vi "LIA Example FPGA.vi"() -> ()   [LabVIEW 2017]
uses:
  <instrlib>/_niInstr/Streaming/v1/Common/Stream State.ctl
  <instrlib>/_niInstr/Data Trigger/v1/Shared/Public/Edge Configuration FXP(+-,18,1).ctl
  <instrlib>/_niInstr/Data Trigger/v1/Shared/Public/Edge Configuration Trigger Slope.ctl
  <vilib>/Platform/TimedLoop/XDataNode/timing_clust.ctl
  <vilib>/Platform/TimedLoop/XDataNode/nitl_modes.ctl
  <vilib>/Platform/TimedLoop/XDataNode/wakeup.ctl
  <instrlib>/_niInstr/DSP/v1/Shared/Public/IQ Data.ctl
  <vilib>/rvi/Emulation/niFpgaSctlEmulationGetInTimedLoop.vi
  <vilib>/rvi/Emulation/niFpgaEmulationReportErrorSimple.vi
  <vilib>/rvi/Emulation/niFpgaGetClockAttributes.vi
  <vilib>/rvi/Emulation/niFpgaCriticalErrorInLSC.vi
  <instrlib>/_niInstr/DSP/v1/FPGA/Public/Sub VIs/Frequency Shift/Frequency Shift - 1 spc.vi
  <userlib>/_NI Noise Generation IP/FPGA/Public/Low Level/AWGN FXP23x2.vi
  <instrlib>/_niInstr/DSP/v1/FPGA/Public/Sub VIs/Frequency Shift/Frequency Shift - 2 spc.vi
  <vilib>/rvi/eio/common/nirviEmuTemplateMethod_errors.vi
  <vilib>/Platform/TimedLoop/XDataNode/XDataNode.xnode
  <instrlib>/_niInstr/DSP/v1/Xnodes/Public/Frequency Shift/niInstr DSP v1 Frequency Shift FPGA.xnode
  <vilib>/rvi/FXPMathLib/FxpMul/XNode/nifxpmath_Multiplier.xnode
  <vilib>/rvi/FXPMathLib/FxpAdd/XNode/nifxpmath_Add.xnode
  <vilib>/eio/EIONode/EIONode.xnode
  <vilib>/Platform/TimedLoop/XDataNode/XDNodeRunTimeDep.lvlib
  <instrlib>/_niInstr/Basic Elements/v1/FPGA/niInstr Basic Elements v1 FPGA.lvlib
  <instrlib>/_niInstr/DSP/v1/Shared/niInstr DSP v1 Shared.lvlib
  <instrlib>/_niInstr/DSP/v1/FPGA/niInstr DSP v1 FPGA.lvlib
  Program Files (x86)/National Instruments/LabVIEW 2017/examples/Lock-In Amplifier/lib/fpga/Lock-In Amplifier Example FPGA.lvlib
  <instrlib>/_niInstr/Streaming/v1/Common/niInstr Streaming v1 Common.lvlib
  <userlib>/_NI Noise Generation IP/FPGA/NI Noise Generation IP FPGA v2.lvlib
  <vilib>/rvi/FXPMathLib/sim/FxpSim.dll
  <instrlib>/_niInstr/Data Trigger/v1/Shared/niInstr Data Trigger v1 Shared.lvlib
panel:
  in  "pll.digital config 1":T1
  in  "pll.digital config 0":T1
  in  "pll.m 0":i8
  in  "pll.m 1":i8
  in  "pll.q 1":fxp<+/-,48,0>
  in  "pll.q 0":fxp<+/-,48,0>
  in  "lock-in.enable 3":bool
  in  "lock-in.enable 2":bool
  in  "lock-in.enable 1":bool
  in  "lock-in.carrier 3":fxp<+/-,48,0>
  in  "lock-in.carrier 2":fxp<+/-,48,0>
  in  "lock-in.enable 0":bool
  in  "lock-in.channel select 3":i32
  in  "lock-in.carrier select 3":i32
  in  "lock-in.cic config valid 3":bool
  in  "lock-in.cic config 3":cluster{"factor":fxp<+,16,16>, "shift":i16}
  in  "lock-in.reset 3":bool
  out "stream.state 3":T3 caption="stream.state 0"
  out "stream.samples transferred 3":u64 caption="stream.samples transferred 0"
  out "stream.metadata 3":u64 caption="stream.metadata 0"
  in  "stream.num samples 3":u64 caption="stream.num samples 0"
  in  "stream.request state 3":T3 caption="stream.request state 0"
  in  "lock-in.channel select 2":i32
  in  "lock-in.carrier select 2":i32
  in  "lock-in.cic config valid 2":bool
  in  "lock-in.cic config 2":cluster{"factor":fxp<+,16,16>, "shift":i16}
  in  "lock-in.reset 2":bool
  out "stream.state 2":T3 caption="stream.state 0"
  out "stream.samples transferred 2":u64 caption="stream.samples transferred 0"
  out "stream.metadata 2":u64 caption="stream.metadata 0"
  in  "stream.num samples 2":u64 caption="stream.num samples 0"
  in  "stream.request state 2":T3 caption="stream.request state 0"
  out "pll.vco output 0":fxp<+/-,48,0> format="%.49g"
  out "pll.vco output 1":fxp<+/-,48,0> format="%.49g"
  out "stream.metadata 4":u64 caption="stream.metadata 0"
  out "stream.samples transferred 4":u64 caption="stream.samples transferred 0"
  out "stream.state 4":T3 caption="stream.state 0"
  in  "stream.request state 4":T3 caption="stream.request state 0"
  in  "stream.num samples 4":u64 caption="stream.num samples 0"
  in  "preview.channel select":i32
  in  "ao.reset 3":bool
  in  "ao.carrier 2":fxp<+/-,48,0>=0.010000000000001563
  in  "ao.level 2":fxp<+/-,18,1>
  in  "ao.reset 2":bool
  in  "ao.carrier 1":fxp<+/-,48,0>=0.010000000000001563
  in  "ao.level 1":fxp<+/-,18,1>
  in  "ao.reset 1":bool
  in  "ao.reset 0":bool
  in  "ao.carrier 0":fxp<+/-,48,0>=0.010000000000001563
  in  "ao.level 0":fxp<+/-,18,1>
  in  "lock-in.channel select 1":i32
  in  "lock-in.channel select 0":i32
  in  "stream.request state 1":T3 caption="stream.request state 0"
  in  "stream.num samples 1":u64 caption="stream.num samples 0"
  out "stream.metadata 1":u64 caption="stream.metadata 0"
  out "stream.samples transferred 1":u64 caption="stream.samples transferred 0"
  out "stream.state 1":T3 caption="stream.state 0"
  in  "lock-in.reset 1":bool
  in  "lock-in.cic config 1":cluster{"factor":fxp<+,16,16>, "shift":i16}
  in  "lock-in.cic config valid 1":bool
  in  "lock-in.carrier select 1":i32
  in  "lock-in.carrier select 0":i32
  in  "lock-in.cic config valid 0":bool
  in  "lock-in.cic config 0":cluster{"factor":fxp<+,16,16>, "shift":i16}
  in  "lock-in.reset 0":bool
  in  "lock-in.carrier 1":fxp<+/-,48,0>
  in  "lock-in.carrier 0":fxp<+/-,48,0>
  in  "ao.level 3":fxp<+/-,18,1>
  in  "pll.channel 1":i32
  in  "pll.reset 1":bool
  in  "pll.enable 1":bool
  in  "pll.channel 0":i32
  in  "ao.noise gain 3":fxp<+,18,1>=0.01000213623046875
  in  "ao.carrier 3":fxp<+/-,48,0>=0.010000000000001563
  in  "ao.noise seeds 3":fxp<+,23,23>[](array[numeric])=[1.0, 12323.0]
  in  "pll.reset 0":bool
  in  "pll.enable 0":bool
  in  "stream.request state 0":T3
  in  "stream.num samples 0":u64
  out "stream.metadata 0":u64
  out "stream.samples transferred 0":u64
  out "stream.state 0":T3
  out "IO Module\\InitDone":bool
  out "IO Module\\User Error":u32
  in  "IO Module\\User Command":u32
  in  "IO Module\\User Command Valid":bool
  out "IO Module\\User Command Ready":bool
  in  "IO Module\\User Command Arg 0":u32
  in  "IO Module\\User Command Arg 1":u32
  out "IO Module\\User Command Error":u16
  out "IO Module\\User Command Return":u32
  out "IO Module\\User Command Return Valid":bool
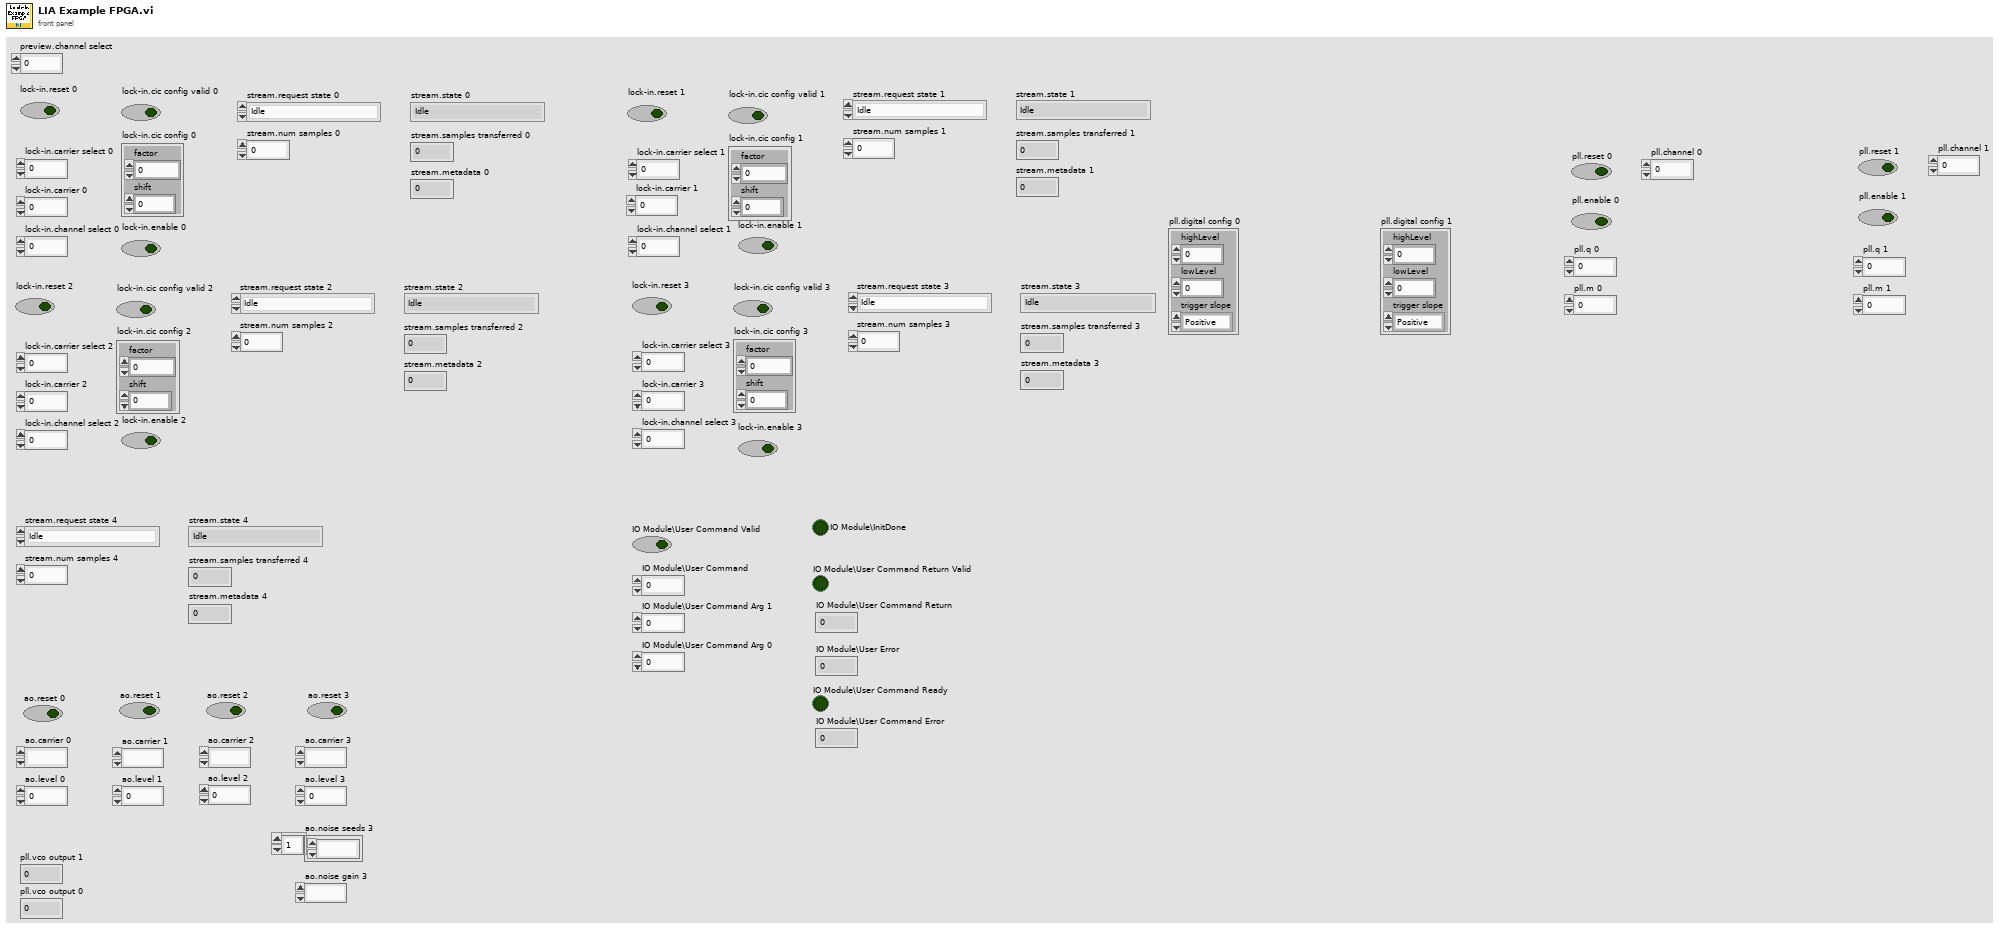
[diagram p1: front panel]
types:
  T1 = typedef "niInstr Data Trigger v1 Shared.lvlib/Edge Configuration FXP(+-,18,1).ctl" = cluster{"highLevel":fxp<+/-,18,1>, "lowLevel":fxp<+/-,18,1>, "trigger slope":T2}
  T2 = typedef "niInstr Data Trigger v1 Shared.lvlib/Edge Configuration Trigger Slope.ctl" = enum8{"Positive", "Negative"}
  T3 = typedef "niInstr Streaming v1 Common.lvlib/Stream State.ctl" = enum8{"Idle", "Finite Transfer", "Continuous", "Done", "Error", "Not Ready", "Cancel"}
  T4 = typedef "XDNodeRunTimeDep.lvlib/timing_clust.ctl" = cluster{"Expected End [f-1]":u64, "Actual End [f-1]":u64, "Finished Late? [f-1]":bool, "Expected End [i-1]":u64, "Actual End [i-1]":u64, "Finished Late? [i-1]":bool, "Expected Start [i]":u64, "Actual Start [i]":u64, "Expected Start [f]":u64, "Actual Start [f]":u64, "Source Name":string, "Structure Name":string, "Period":i64, "Deadline":i64, "Offset":i64, "Start":i64, "Priority":i32, "Timeout":i32, "Mode":T5, "Wakeup Reason":T6, "Error":errorcluster, "Source Type":string, "Secondary Source Type":string, "Global End Time":u64, "Global Start Time":u64, "Frame Duration":u64, "Iteration Duration":u64, "Assigned CPU":i32, "I/O Scan Engine Mode":u32}
  T5 = typedef "XDNodeRunTimeDep.lvlib/nitl_modes.ctl" = enum32{"No Change", "Process missed periods, maintain original phase", "Discard missed periods, maintain original phase", "Process missed periods, ignore original phase", "Discard missed periods, ignore original phase"}
  T6 = typedef "XDNodeRunTimeDep.lvlib/wakeup.ctl" = enum32{"Normal", "Aborted", "Asynchronous wakeup", "Timing source error", "Timed loop error", "Timeout"}
  T7 = cluster{"stream.num samples 0":u64, "stream.request state 0":T3, "stream.index 0":i16}
  T8 = typedef "niInstr DSP v1 Shared.lvlib/IQ Data.ctl" = cluster{"I":fxp<+/-,18,1>, "Q":fxp<+/-,18,1>, "overflow":bool}
  T9 = cluster{"stream.metadata 0":u64, "stream.samples transferred 0":u64, "stream.state 0":T3}
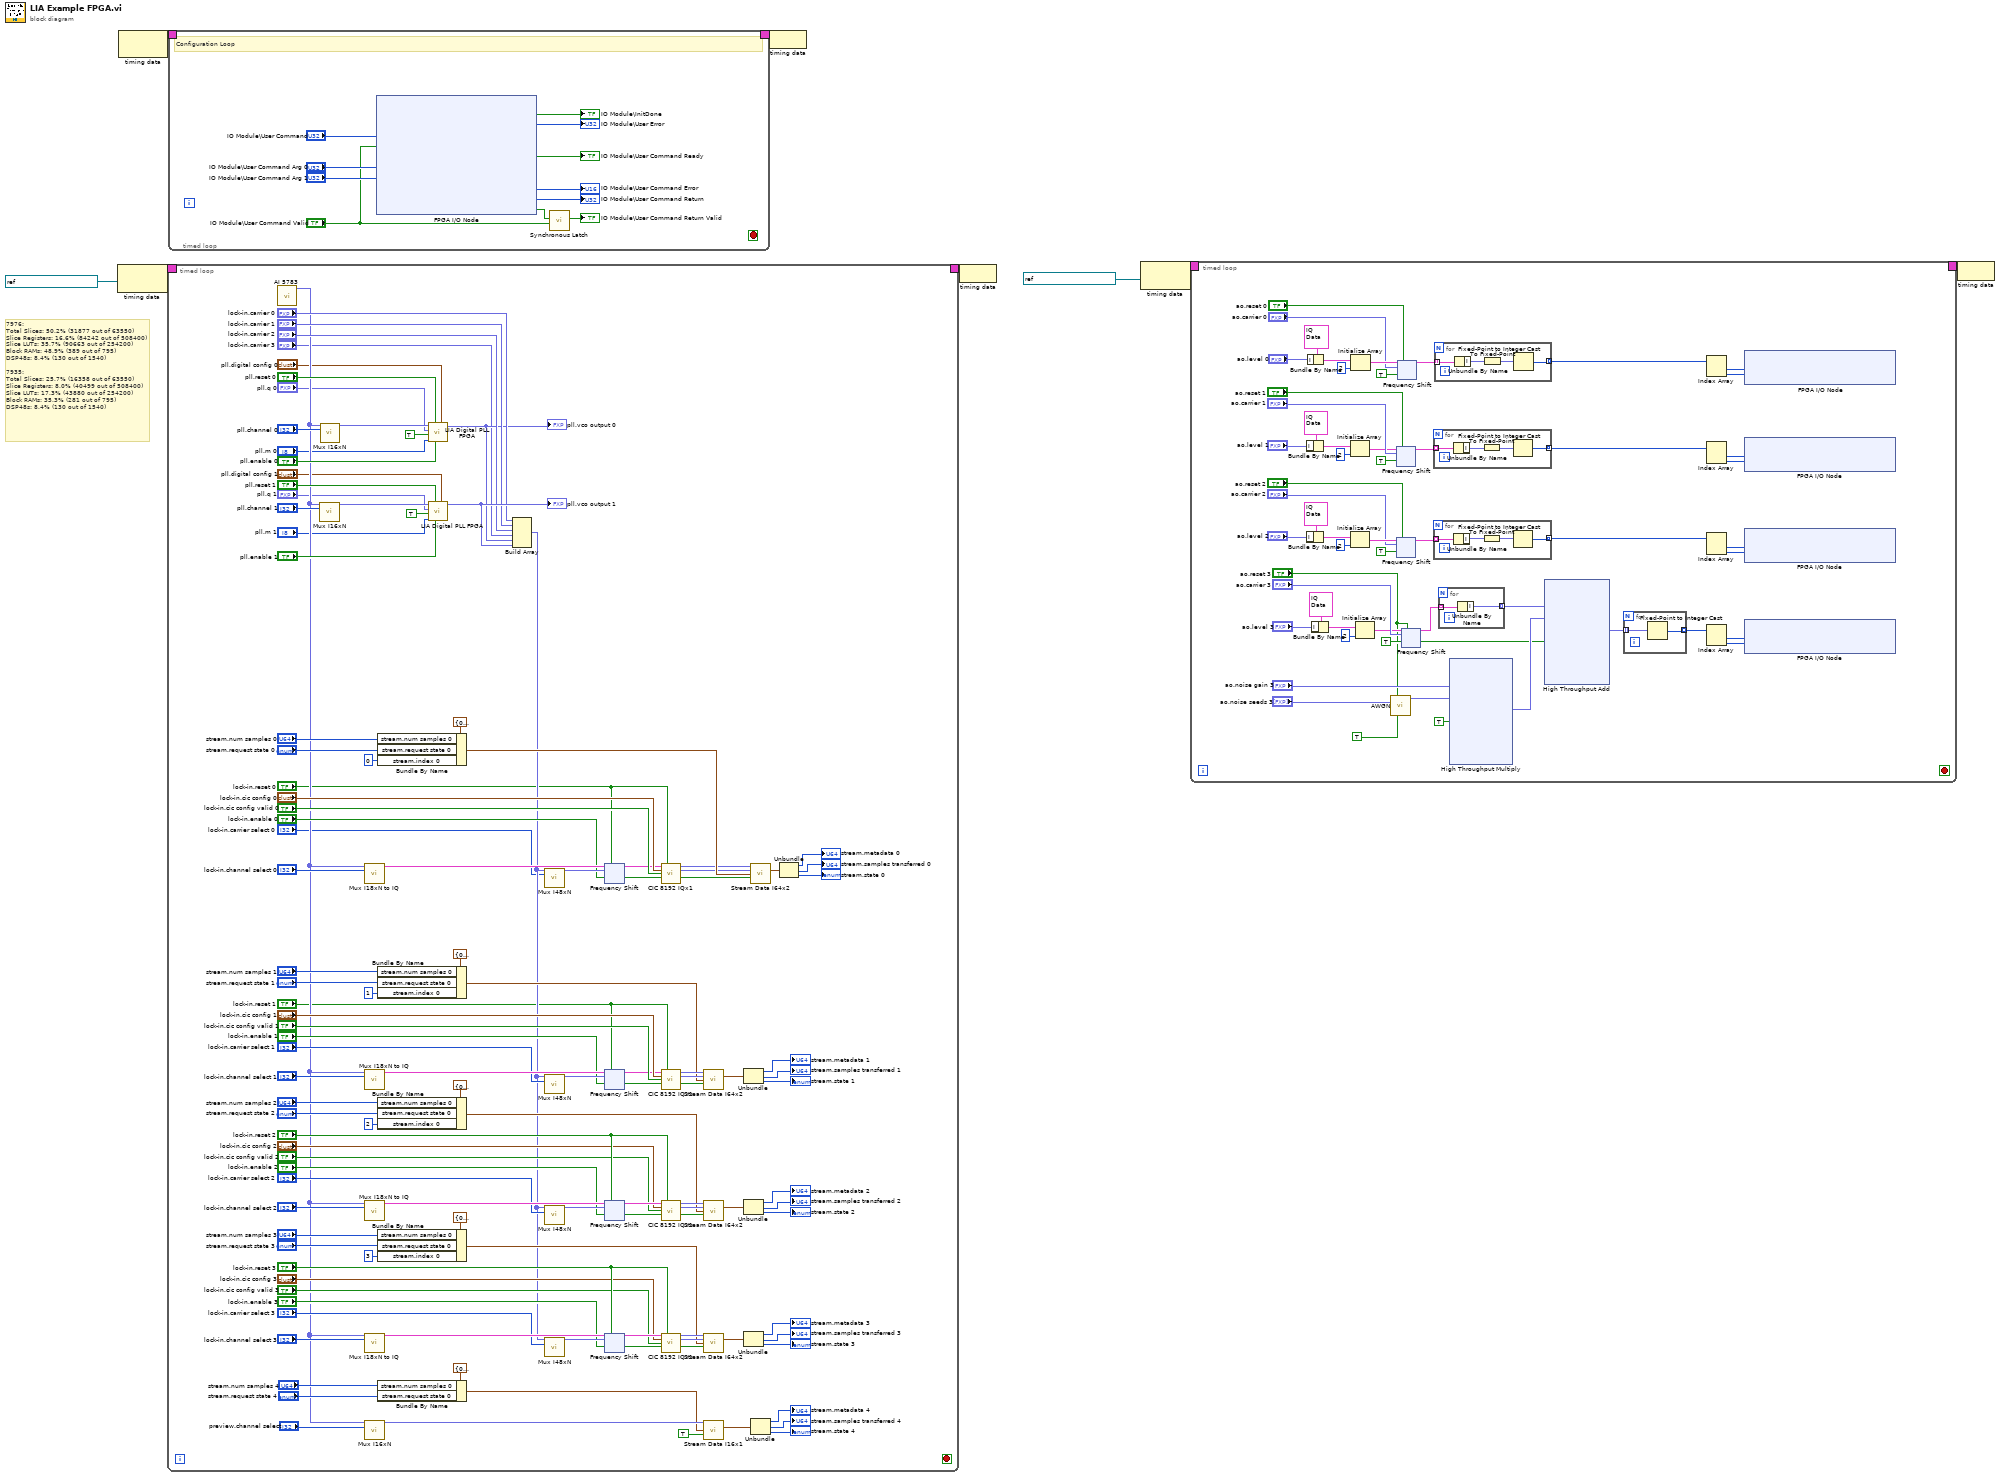
[diagram p0: block diagram]
diagram:
  # "7976:\nTotal Slices: 50.2% (31877 out of 63550)\nSlice Registers: 16.6% (84242 out of 508400)\nSlice LUTs: 35.7% (90663 out of 254200)\nBlock RAMs: 48.9% (389 out of 795)\nDSP48s: 8.4% (130 out of 1540)\n\n7935:\nTotal Slices: 25.7% (16358 out of 63550)\nSlice Registers: 8.0% (40499 out of 508400)\nSlice LUTs: 17.3% (43880 out of 254200)\nBlock RAMs: 35.3% (281 out of 795)\nDSP48s: 8.4% (130 out of 1540)"
  n1 = node-c288(refnum<k21> "IO Module\\Data Clock" ("Source Name")) -> (w8:T4)
  n2 = node-c288() -> (w2:T4)  [unwired: 1 in]
  n3 = timed-loop {
    timing: w8 -> [_]
    timing-out: [_] -> w7
    stop <- _ stop-if-true
    n4 = call "AI 5783.vi"() -> ("i18x1"=w27:fxp<+/-,18,1>[])  [unwired: 14 in, 1 out]
    n5 = call "Mux I16xN.vi"("i16xn in"=w27, "index"="pll.channel 1") -> ("i16 out"=w30:fxp<+/-,18,1>)  [unwired: 12 in, 1 out]
    n6 = call "Mux I16xN.vi"("i16xn in"=w27, "index"="pll.channel 0") -> ("i16 out"=w129:fxp<+/-,18,1>)  [unwired: 12 in, 1 out]
    n7 = call "Mux I18xN to IQ.vi"("i16xn in"=w27, "index"="lock-in.channel select 0") -> ("output"=w124:T8)  [unwired: 12 in, 1 out]
    n8 = call "Mux I18xN to IQ.vi"("i16xn in"=w27, "index"="lock-in.channel select 1") -> ("output"=w110:T8)  [unwired: 12 in, 1 out]
    n9 = call "Mux I18xN to IQ.vi"("i16xn in"=w27, "index"="lock-in.channel select 2") -> ("output"=w81:T8)  [unwired: 12 in, 1 out]
    n10 = call "Mux I18xN to IQ.vi"("i16xn in"=w27, "index"="lock-in.channel select 3") -> ("output"=w60:T8)  [unwired: 12 in, 1 out]
    n11 = call "Mux I16xN.vi"("i16xn in"=w27, "index"="preview.channel select") -> ("i16 out"=w87:fxp<+/-,18,1>)  [unwired: 12 in, 1 out]
    n12 = Bundle By Name(cluster=T7 {"stream.num samples 0"=0, "stream.request state 0"=enum."Idle", "stream.index 0"=0} ("config"), "stream.num samples 0"="stream.num samples 0", "stream.request state 0"="stream.request state 0", "stream.index 0"=i16 0) -> (w112:T7)
    n13 = Bundle By Name(cluster=T7 {"stream.num samples 0"=0, "stream.request state 0"=enum."Idle", "stream.index 0"=0} ("config"), "stream.num samples 0"="stream.num samples 1", "stream.request state 0"="stream.request state 1", "stream.index 0"=i16 1) -> (w95:T7)
    n14 = Bundle By Name(cluster=T7 {"stream.num samples 0"=0, "stream.request state 0"=enum."Idle", "stream.index 0"=0} ("config"), "stream.num samples 0"="stream.num samples 2", "stream.request state 0"="stream.request state 2", "stream.index 0"=i16 2) -> (w63:T7)
    n15 = Bundle By Name(cluster=T7 {"stream.num samples 0"=0, "stream.request state 0"=enum."Idle", "stream.index 0"=0} ("config"), "stream.num samples 0"="stream.num samples 3", "stream.request state 0"="stream.request state 3", "stream.index 0"=i16 3) -> (w42:T7)
    n16 = Bundle By Name(cluster=T7 {"stream.num samples 0"=0, "stream.request state 0"=enum."Idle", "stream.index 0"=0} ("config"), "stream.num samples 0"="stream.num samples 4", "stream.request state 0"="stream.request state 4") -> (w84:T7)
    n17 = call "LIA Digital PLL FPGA.vi"("configuration"="pll.digital config 0", "arm"="pll.enable 0", "reset"="pll.reset 0", "m"="pll.m 0", "input valid"=TRUE ("output valid"), "q"="pll.q 0", "I"=w129) -> ("frequency shift"=w29:fxp<+/-,48,0>)  [unwired: 1 in, 3 out]
    "pll.vco output 0" <- w29
    n18 = call "LIA Digital PLL FPGA.vi"("configuration"="pll.digital config 1", "arm"="pll.enable 1", "reset"="pll.reset 1", "m"="pll.m 1", "input valid"=TRUE ("output valid"), "q"="pll.q 1", "I"=w30) -> ("frequency shift"=w82:fxp<+/-,48,0>)  [unwired: 1 in, 3 out]
    "pll.vco output 1" <- w82
    n19 = Build Array("lock-in.carrier 0", "lock-in.carrier 1", "lock-in.carrier 2", "lock-in.carrier 3", w29, w82) -> (w28:fxp<+/-,48,0>[])
    n20 = call "Mux I48xN.vi"("i48xn in"=w28, "index"="lock-in.carrier select 0") -> ("i48 out"=w123:fxp<+/-,48,0>)  [unwired: 13 in]
    n21 = call "Mux I48xN.vi"("i48xn in"=w28, "index"="lock-in.carrier select 1") -> ("i48 out"=w109:fxp<+/-,48,0>)  [unwired: 13 in]
    n22 = call "Mux I48xN.vi"("i48xn in"=w28, "index"="lock-in.carrier select 2") -> ("i48 out"=w80:fxp<+/-,48,0>)  [unwired: 13 in]
    n23 = call "Mux I48xN.vi"("i48xn in"=w28, "index"="lock-in.carrier select 3") -> ("i48 out"=w59:fxp<+/-,48,0>)  [unwired: 13 in]
    n24 = xnode "Frequency Shift"("data in"=w124, "reset"="lock-in.reset 0", "frequency shift"=w123, "input valid"="lock-in.enable 0") -> ("data out"=w13:T8, "output valid"=w12:bool)  [unwired: 2 in, 1 out]
    n25 = xnode "Frequency Shift"("data in"=w110, "reset"="lock-in.reset 1", "frequency shift"=w109, "input valid"="lock-in.enable 1") -> ("data out"=w17:T8, "output valid"=w16:bool)  [unwired: 2 in, 1 out]
    n26 = xnode "Frequency Shift"("data in"=w81, "reset"="lock-in.reset 2", "frequency shift"=w80, "input valid"="lock-in.enable 2") -> ("data out"=w79:T8, "output valid"=w78:bool)  [unwired: 2 in, 1 out]
    n27 = xnode "Frequency Shift"("data in"=w60, "reset"="lock-in.reset 3", "frequency shift"=w59, "input valid"="lock-in.enable 3") -> ("data out"=w58:T8, "output valid"=w57:bool)  [unwired: 2 in, 1 out]
    n28 = call "CIC 8192 IQx1.vi"("data"=w13, "reset"="lock-in.reset 0", "config"="lock-in.cic config 0", "config valid"="lock-in.cic config valid 0", "input valid"=w12) -> ("i out"=w11:fxp<+/-,64,1>, "q out"=w10:fxp<+/-,64,1>, "output valid"=w9:bool)  [unwired: 8 in]
    n29 = call "CIC 8192 IQx1.vi"("data"=w17, "reset"="lock-in.reset 1", "config"="lock-in.cic config 1", "config valid"="lock-in.cic config valid 1", "input valid"=w16) -> ("i out"=w106:fxp<+/-,64,1>, "q out"=w105:fxp<+/-,64,1>, "output valid"=w104:bool)  [unwired: 8 in]
    n30 = call "CIC 8192 IQx1.vi"("data"=w79, "reset"="lock-in.reset 2", "config"="lock-in.cic config 2", "config valid"="lock-in.cic config valid 2", "input valid"=w78) -> ("i out"=w74:fxp<+/-,64,1>, "q out"=w73:fxp<+/-,64,1>, "output valid"=w72:bool)  [unwired: 8 in]
    n31 = call "CIC 8192 IQx1.vi"("data"=w58, "reset"="lock-in.reset 3", "config"="lock-in.cic config 3", "config valid"="lock-in.cic config valid 3", "input valid"=w57) -> ("i out"=w53:fxp<+/-,64,1>, "q out"=w52:fxp<+/-,64,1>, "output valid"=w51:bool)  [unwired: 8 in]
    n32 = call "Stream Data I64x2.vi"("i in"=w106, "q in"=w105, "config"=w95, "input valid"=w104) -> ("status"=w103:T9)  [unwired: 11 in]
    n33 = call "Stream Data I64x2.vi"("i in"=w74, "q in"=w73, "config"=w63, "input valid"=w72) -> ("status"=w71:T9)  [unwired: 11 in]
    n34 = call "Stream Data I64x2.vi"("i in"=w53, "q in"=w52, "config"=w42, "input valid"=w51) -> ("status"=w50:T9)  [unwired: 11 in]
    n35 = call "Stream Data I16x1.vi"("i in"=w87, "config"=w84, "input valid"=TRUE) -> ("status"=w89:T9)  [unwired: 12 in]
    n36 = Unbundle(w103) -> ("stream.metadata 0"=→"stream.metadata 1":u64, "stream.samples transferred 0"=→"stream.samples transferred 1":u64, "stream.state 0"=→"stream.state 1":T3)
    n37 = Unbundle(w71) -> ("stream.metadata 0"=→"stream.metadata 2":u64, "stream.samples transferred 0"=→"stream.samples transferred 2":u64, "stream.state 0"=→"stream.state 2":T3)
    n38 = Unbundle(w50) -> ("stream.metadata 0"=→"stream.metadata 3":u64, "stream.samples transferred 0"=→"stream.samples transferred 3":u64, "stream.state 0"=→"stream.state 3":T3)
    n39 = call "Stream Data I64x2.vi"("i in"=w11, "q in"=w10, "config"=w112, "input valid"=w9) -> ("status"=w120:T9)  [unwired: 11 in]
    n40 = Unbundle(w89) -> ("stream.metadata 0"=→"stream.metadata 4":u64, "stream.samples transferred 0"=→"stream.samples transferred 4":u64, "stream.state 0"=→"stream.state 4":T3)
    n41 = Unbundle(w120) -> ("stream.metadata 0"=→"stream.metadata 0":u64, "stream.samples transferred 0"=→"stream.samples transferred 0":u64, "stream.state 0"=→"stream.state 0":T3)
  }
  n42 = timed-loop {
    timing: w2 -> [_]
    timing-out: [_] -> w1
    stop <- _ stop-if-true
    # "Configuration Loop"
    n43 = xnode "FPGA I/O Node"("IO Module\\User Command"="IO Module\\User Command", "IO Module\\User Command Valid"="IO Module\\User Command Valid", "IO Module\\User Command Arg 0"="IO Module\\User Command Arg 0", "IO Module\\User Command Arg 1"="IO Module\\User Command Arg 1") -> ("IO Module\\InitDone"=→"IO Module\\InitDone":bool, "IO Module\\Clip Error Code"=→"IO Module\\User Error":u32, "IO Module\\User Command Ready"=→"IO Module\\User Command Ready":bool, "IO Module\\User Command Error"=→"IO Module\\User Command Error":u16, "IO Module\\User Command Return"=→"IO Module\\User Command Return":u32, "IO Module\\User Command Return Valid"=w171:bool)  [unwired: 10 in, 10 out]
    n44 = call <instrlib>:"Synchronous Latch.vi"("clear"="IO Module\\User Command Valid", "set"=w171) -> ("out"=→"IO Module\\User Command Return Valid":bool)  [unwired: 9 in]
  }
  n45 = node-c288(w1) -> ()
  n46 = node-c288(w7) -> ()
  n47 = node-c288(refnum<k21> "IO Module\\Data Clock" ("Source Name")) -> (w5:T4)
  n48 = timed-loop {
    timing: w5 -> [_]
    timing-out: [_] -> w4
    stop <- _ stop-if-true
    n49 = Bundle By Name(cluster=T8 {"I"=0.0, "Q"=0.0, "overflow"=FALSE} ("output"), "I"="ao.level 1") -> (w204:T8)
    n50 = Bundle By Name(cluster=T8 {"I"=0.0, "Q"=0.0, "overflow"=FALSE} ("output"), "I"="ao.level 2") -> (w194:T8)
    n51 = Bundle By Name(cluster=T8 {"I"=0.0, "Q"=0.0, "overflow"=FALSE} ("output"), "I"="ao.level 0") -> (w219:T8)
    n52 = Bundle By Name(cluster=T8 {"I"=0.0, "Q"=0.0, "overflow"=FALSE} ("output"), "I"="ao.level 3") -> (w228:T8)
    n53 = Initialize Array(w204, 2 ("dimension size")) -> (w200:T8[])
    n54 = Initialize Array(w194, 2 ("dimension size")) -> (w198:T8[])
    n55 = Initialize Array(w219, 2 ("dimension size")) -> (w223:T8[])
    n56 = Initialize Array(w228, 2 ("dimension size")) -> (w224:T8[])
    n57 = call-poly <userlib>:"AWGN.vi"("reset"="ao.reset 3", "seeds"="ao.noise seeds 3", "ready"=TRUE) -> ("output 0"=w231:fxp<+/-,23,4>[])  [unwired: 10 in, 2 out]
    n58 = xnode "Frequency Shift"("data in"=w200, "reset"="ao.reset 1", "frequency shift"="ao.carrier 1", "input valid"=TRUE) -> ("data out"=w208:T8[])  [unwired: 2 in, 2 out]
    n59 = xnode "Frequency Shift"("data in"=w198, "reset"="ao.reset 2", "frequency shift"="ao.carrier 2", "input valid"=TRUE) -> ("data out"=w190:T8[])  [unwired: 2 in, 2 out]
    n60 = xnode "Frequency Shift"("data in"=w223, "reset"="ao.reset 0", "frequency shift"="ao.carrier 0", "input valid"=TRUE) -> ("data out"=w215:T8[])  [unwired: 2 in, 2 out]
    n61 = xnode "Frequency Shift"("data in"=w224, "reset"="ao.reset 3", "frequency shift"="ao.carrier 3", "input valid"=TRUE) -> ("data out"=w239:T8[], "output valid"=w236:bool)  [unwired: 2 in, 1 out]
    n62 = for {
      tunnel: w208 -> [w255] mode=indexing
      tunnel: [w256] -> w209 mode=indexing
      n63 = Unbundle By Name(w255) -> ("I"=w254:fxp<+/-,18,1>)
      n64 = To Fixed-Point(number=w254) -> (fixed-point=w253:fxp<+/-,16,1>)  [unwired: 1 in]
      n65 = Fixed-Point to Integer Cast(1:w253) -> (0:w256:i16)
    }
    n66 = for {
      tunnel: w190 -> [w242] mode=indexing
      tunnel: [w243] -> w189 mode=indexing
      n67 = Unbundle By Name(w242) -> ("I"=w241:fxp<+/-,18,1>)
      n68 = To Fixed-Point(number=w241) -> (fixed-point=w240:fxp<+/-,16,1>)  [unwired: 1 in]
      n69 = Fixed-Point to Integer Cast(1:w240) -> (0:w243:i16)
    }
    n70 = for {
      tunnel: w215 -> [w268] mode=indexing
      tunnel: [w269] -> w214 mode=indexing
      n71 = Unbundle By Name(w268) -> ("I"=w267:fxp<+/-,18,1>)
      n72 = To Fixed-Point(number=w267) -> (fixed-point=w266:fxp<+/-,16,1>)  [unwired: 1 in]
      n73 = Fixed-Point to Integer Cast(1:w266) -> (0:w269:i16)
    }
    n74 = for {
      tunnel: w239 -> [w282] mode=indexing
      tunnel: [w281] -> w235 mode=indexing
      n75 = Unbundle By Name(w282) -> ("I"=w281:fxp<+/-,18,1>)
    }
    n76 = xnode ("High Throughput Multiply")("x"="ao.noise gain 3", "y"=w231, "input valid"=TRUE) -> ("x*y"=w238:fxp<+/-,41,5>[])  [unwired: 1 in, 2 out]
    n77 = xnode ("High Throughput Add")("x"=w235, "y"=w238, "input valid"=w236) -> ("x+y"=w230:fxp<+/-,16,1>[])  [unwired: 1 in, 2 out]
    n78 = for {
      tunnel: w230 -> [w280] mode=indexing
      tunnel: [w279] -> w199 mode=indexing
      n79 = Fixed-Point to Integer Cast(1:w280) -> (0:w279:i16)
    }
    n80 = Index Array(array=w214) -> (element #1=w213:i16, element #2=w212:i16)  [unwired: 2 in]
    n81 = Index Array(array=w209) -> (element #1=w210:i16, element #2=w211:i16)  [unwired: 2 in]
    n82 = Index Array(array=w189) -> (element #1=w188:i16, element #2=w187:i16)  [unwired: 2 in]
    n83 = Index Array(array=w199) -> (element #1=w186:i16, element #2=w185:i16)  [unwired: 2 in]
    n84 = xnode "FPGA I/O Node"("IO Module\\AO 1 Data N-1 Data Clock"=w210, "IO Module\\AO 1 Data N Data Clock"=w211) -> ()  [unwired: 2 in, 2 out]
    n85 = xnode "FPGA I/O Node"("IO Module\\AO 2 Data N-1 Data Clock"=w188, "IO Module\\AO 2 Data N Data Clock"=w187) -> ()  [unwired: 2 in, 2 out]
    n86 = xnode "FPGA I/O Node"("IO Module\\AO 3 Data N-1 Data Clock"=w186, "IO Module\\AO 3 Data N Data Clock"=w185) -> ()  [unwired: 2 in, 2 out]
    n87 = xnode "FPGA I/O Node"("IO Module\\AO 0 Data N-1 Data Clock"=w213, "IO Module\\AO 0 Data N Data Clock"=w212) -> ()  [unwired: 2 in, 2 out]
  }
  n88 = node-c288(w4) -> ()
